vi "Fetch (Waveform).vi"(7 "Segment Index (0)":i32 format="%.0g", 8 "error in (no error)":errorcluster, 9 "Maximum Time (10000ms)":u32, 10 "Channel (1: Channel 1)":i32(ring) items=["Channel 1", "Channel 2", "Channel 3", "Channel 4", "Function 1", "Function 2", "Function 3", "Function 4", "Memory 1", "Memory 2", "Memory 3", "Memory 4"], 11 "VISA resource name":refnum<visa-resource-name>) -> (0 "error out":errorcluster, 2 "Waveform Data":waveform(dbl)(graph), 3 "VISA resource name out":refnum<visa-resource-name>)   [LabVIEW 2009, in "Agilent 8000 Series.lvlib"]
doc: "Returns the waveform the oscilloscope acquired for the specified channel. The waveform is from an acquisition that you initiate prior to calling this VI.\n\nYou use the Initiate VI to start an acquisition on the channels that you enable with the Configure Channel VI. The oscilloscope acquires waveforms for the enabled channels concurrently. You must call this VI separately for each enabled channel to obtain the waveforms.\n\nYou can call the Read Waveform VI instead of using low-level VIs.\n\n<B>Note:</B> Use this VI only with other low-level VIs. The high-level VIs automatically incorporate this functionality. This VI does not check the instrument status."
uses:
  Agilent 8000 Series.lvlib
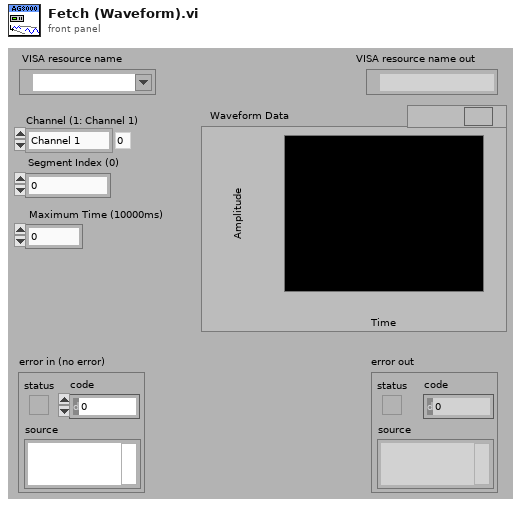
[diagram p1: front panel]
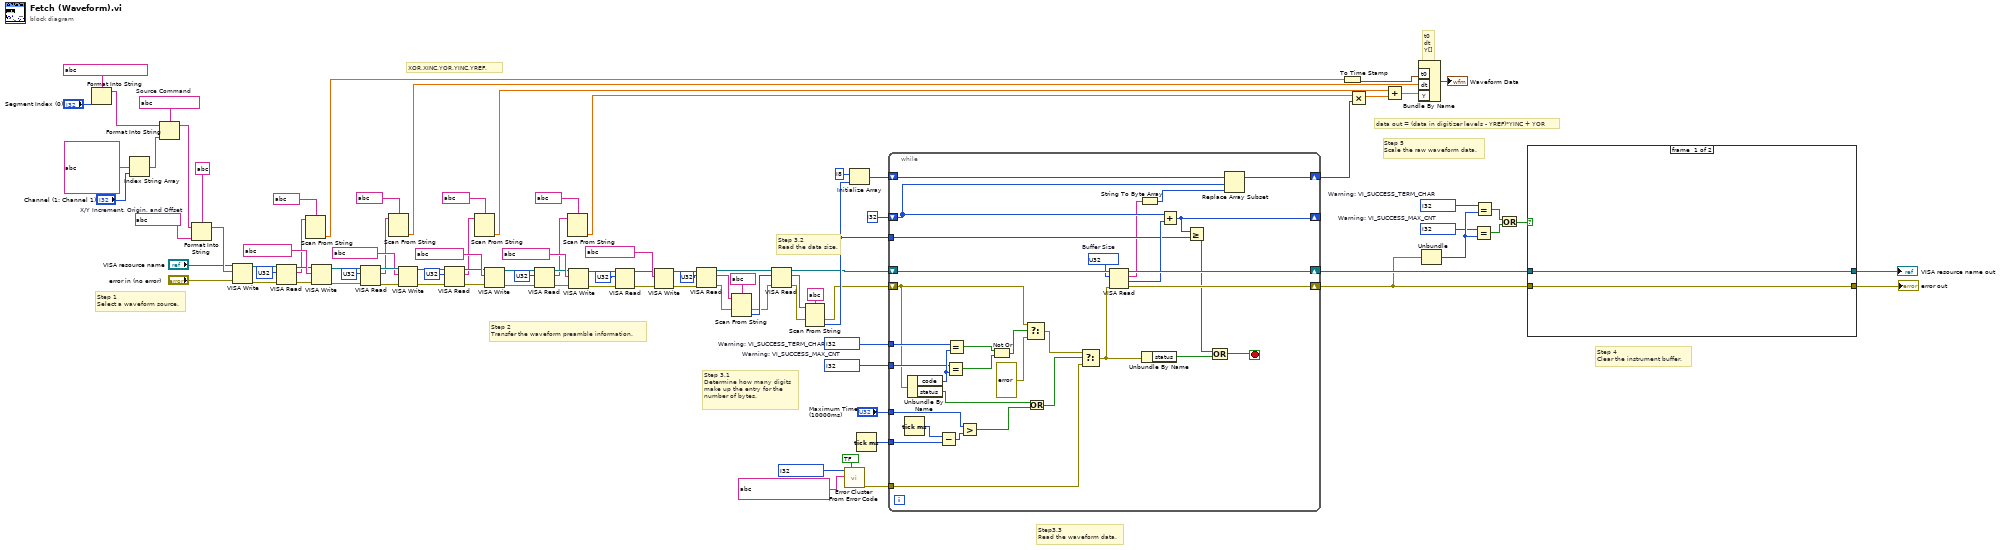
[diagram p0: block diagram]
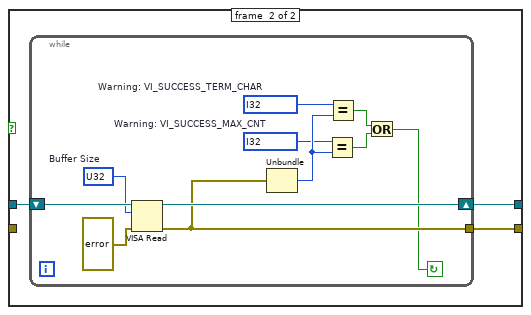
[diagram p2: hidden frame]
diagram:
  w69 = i32 ?  # Warning: VI_SUCCESS_MAX_CNT
  w68 = i32 ?  # Warning: VI_SUCCESS_TERM_CHAR
  w61 = i32 ?  # Warning: VI_SUCCESS_MAX_CNT
  w60 = i32 ?  # Warning: VI_SUCCESS_TERM_CHAR
  w91 = string ?  # Source Command
  w82 = string ?  # X/Y Increment, Origin, and Offset
  # "Step 5    \nScale the raw waveform data."
  # "Step 4    \nClear the instrument buffer."
  # "Step3.3   \nRead the waveform data."
  # "Step 3.2     \nRead the data size."
  # "Step 3.1     \nDetermine how many digits\nmake up the entry for the \nnumber of bytes."
  # "Step 2\nTransfer the waveform preamble information."
  # "Step 1       \nSelect a waveform source."
  # "XOR,XINC,YOR,YINC,YREF,"
  # "data out = (data in digitizer levels - YREF)*YINC + YOR"
  # "t0\ndt\nY[]"
  n1 = Format Into String(format string=string ?, "Segment Index (0)") -> (resulting string=w77:string)  [unwired: 2 in, 1 out]
  n2 = Index String Array(1:"Channel (1: Channel 1)", 2:string[] ?) -> (0:w83:string)  [unwired: 1 in]
  n3 = Format Into String(format string=w91, initial string=w77, w83) -> (resulting string=w89:string)  [unwired: 1 in, 1 out]
  n4 = Format Into String(format string=string ?, initial string=w89, w82) -> (resulting string=w88:string)  [unwired: 1 in, 1 out]
  n5 = VISA Write(VISA resource name="VISA resource name", write buffer=w88, error in (no error)="error in (no error)") -> (VISA resource name out=w96:refnum<visa-resource-name>, error out=w95:errorcluster)  [unwired: 1 out]
  n6 = VISA Read(VISA resource name=w96, byte count=u32 ?, error in (no error)=w95) -> (VISA resource name out=w31:refnum<visa-resource-name>, read buffer=w8:string, error out=w30:errorcluster)  [unwired: 1 out]
  n7 = Scan From String(format string=string ?, input string=w8) -> (output 1=w4:dbl)  [unwired: 3 in, 3 out]
  n8 = VISA Write(VISA resource name=w31, write buffer=string ?, error in (no error)=w30) -> (VISA resource name out=w29:refnum<visa-resource-name>, error out=w28:errorcluster)  [unwired: 1 out]
  n9 = VISA Read(VISA resource name=w29, byte count=u32 ?, error in (no error)=w28) -> (VISA resource name out=w27:refnum<visa-resource-name>, read buffer=w7:string, error out=w26:errorcluster)  [unwired: 1 out]
  n10 = Scan From String(format string=string ?, input string=w7) -> (output 1=w3:dbl)  [unwired: 3 in, 3 out]
  n11 = VISA Write(VISA resource name=w27, write buffer=string ?, error in (no error)=w26) -> (VISA resource name out=w25:refnum<visa-resource-name>, error out=w24:errorcluster)  [unwired: 1 out]
  n12 = VISA Read(VISA resource name=w25, byte count=u32 ?, error in (no error)=w24) -> (VISA resource name out=w23:refnum<visa-resource-name>, read buffer=w6:string, error out=w22:errorcluster)  [unwired: 1 out]
  n13 = Scan From String(format string=string ?, input string=w6) -> (output 1=w2:dbl)  [unwired: 3 in, 3 out]
  n14 = VISA Write(VISA resource name=w23, write buffer=string ?, error in (no error)=w22) -> (VISA resource name out=w21:refnum<visa-resource-name>, error out=w20:errorcluster)  [unwired: 1 out]
  n15 = VISA Read(VISA resource name=w21, byte count=u32 ?, error in (no error)=w20) -> (VISA resource name out=w19:refnum<visa-resource-name>, read buffer=w5:string, error out=w18:errorcluster)  [unwired: 1 out]
  n16 = Scan From String(format string=string ?, input string=w5) -> (output 1=w1:dbl)  [unwired: 3 in, 3 out]
  n17 = VISA Write(VISA resource name=w19, write buffer=string ?, error in (no error)=w18) -> (VISA resource name out=w17:refnum<visa-resource-name>, error out=w16:errorcluster)  [unwired: 1 out]
  n18 = VISA Read(VISA resource name=w17, byte count=u32 ?, error in (no error)=w16) -> (VISA resource name out=w15:refnum<visa-resource-name>, error out=w14:errorcluster)  [unwired: 2 out]
  n19 = VISA Write(VISA resource name=w15, write buffer=string ?, error in (no error)=w14) -> (VISA resource name out=w44:refnum<visa-resource-name>, error out=w43:errorcluster)  [unwired: 1 out]
  n20 = VISA Read(VISA resource name=w44, byte count=u32 ?, error in (no error)=w43) -> (VISA resource name out=w50:refnum<visa-resource-name>, read buffer=w47:string, error out=w46:errorcluster)  [unwired: 1 out]
  n21 = Scan From String(format string=string ?, input string=w47, error in=w46) -> (error out=w49:errorcluster, output 1=w76:i32)  [unwired: 2 in, 2 out]
  n22 = VISA Read(VISA resource name=w50, byte count=w76, error in (no error)=w49) -> (VISA resource name out=w54:refnum<visa-resource-name>, read buffer=w53:string, error out=w51:errorcluster)  [unwired: 1 out]
  n23 = Scan From String(format string=string ?, input string=w53, error in=w51) -> (error out=w55:errorcluster, output 1=w59:i32)  [unwired: 2 in, 2 out]
  n24 = call <vilib>:"Error Cluster From Error Code.vi"("show call chain? (False)"=bool ?, "error message (\"\")"=string ? ("error message (\"\")"), "error code (0)"=i32 ?) -> ("error out"=w67:errorcluster)  [unwired: 6 in]
  n25 = Initialize Array(i8 ? ("element"), w59) -> (w57:i8[])
  n26 = Tick Count (ms)() -> (millisecond timer value=w66:u32)
  n27 = while {
    shift-right: [w124] -> w74
    shift-left: w55 -> [w111]
    shift-right: [w129] -> w75
    shift-left: w54 -> [w128]
    shift-right: [w125] -> w39
    shift-left: w57 -> [w126]
    shift-right: [w121] -> _
    shift-left: i32 ? ("index") -> [w122]
    tunnel: w59 -> [w120]
    tunnel: w60 -> [w113]
    tunnel: w61 -> [w112]
    tunnel: "Maximum Time (10000ms)" -> [w108]
    tunnel: w66 -> [w107]
    tunnel: w67 -> [w102]
    stop <- w99 stop-if-true
    w127 = u32 ?  # Buffer Size
    n28 = Tick Count (ms)() -> (millisecond timer value=w109:u32)
    n29 = Unbundle By Name(w111) -> ("code"=w114:i32, "status"=w106:bool)
    n30 = Subtract(x=w109, y=w107) -> (x-y=w110:u32)
    n31 = Equal?(x=w112, y=w114) -> (x = y?=w117:bool)
    n32 = Equal?(x=w113, y=w114) -> (x = y?=w118:bool)
    n33 = Greater?(x=w108, y=w110) -> (0:w105:bool)
    n34 = Not Or(1:w117, 2:w118) -> (0:w116:bool)
    n35 = Select(t=w111, s=w116, f=errorcluster ? ("error in (no error)")) -> (s? t:f=w104:errorcluster)
    n36 = Or(x=w106, y=w105) -> (x .or. y?=w103:bool)
    n37 = Select(t=w104, s=w103, f=w102) -> (s? t:f=w101:errorcluster)
    n38 = VISA Read(VISA resource name=w128, byte count=w127, error in (no error)=w101) -> (VISA resource name out=w129:refnum<visa-resource-name>, read buffer=w98:string, return count=w123:u32, error out=w124:errorcluster)
    n39 = String To Byte Array(string=w98) -> (unsigned byte array=w97:u8[])
    n40 = Unbundle By Name(w101) -> ("status"=w100:bool)
    n41 = Add(x=w122, y=w123) -> (x+y=w121:u32)
    n42 = Greater Or Equal?(x=w121, y=w120) -> (x >= y?=w119:bool)
    n43 = Compound Arithmetic op=OR(w119, w100) -> (w99:bool)
    n44 = Replace Array Subset(array=w126, new element=w97, index=w122) -> (w125:i8[])
  }
  n45 = To Time Stamp(1:w4) -> (0:w93:timestamp)
  n46 = Multiply(x=w1, y=w39) -> (x*y=w86:dbl[])
  n47 = Add(x=w2, y=w86) -> (x+y=w87:dbl[])
  n48 = Bundle By Name("t0"=w93, "dt"=w3, "Y"=w87) -> (→"Waveform Data":waveform(dbl))  [unwired: 1 in]
  n49 = Unbundle(w74) -> ("code"=w70:i32)  [unwired: 2 out]
  n50 = Equal?(x=w69, y=w70) -> (x = y?=w72:bool)
  n51 = Equal?(x=w68, y=w70) -> (x = y?=w73:bool)
  n52 = Or(x=w73, y=w72) -> (x .or. y?=w71:bool)
  n53 = case shown="True" w71 {
    tunnel: w75 -> [w131 w134]
    tunnel: w74 -> [w130 _]
    tunnel: [w131 w133] -> w41
    tunnel: [w130 w132] -> w40
    frame #0 {
    }
    frame #1 {
      n54 = while {
        shift-right: [w144] -> w133
        shift-left: w134 -> [w145]
        tunnel: [w137] -> w132
        stop <- w136 continue-if-true
        w139 = i32 ?  # Warning: VI_SUCCESS_MAX_CNT
        w138 = i32 ?  # Warning: VI_SUCCESS_TERM_CHAR
        w143 = u32 ?  # Buffer Size
        n55 = VISA Read(VISA resource name=w145, byte count=w143, error in (no error)=errorcluster ?) -> (VISA resource name out=w144:refnum<visa-resource-name>, error out=w137:errorcluster)  [unwired: 2 out]
        n56 = Unbundle(w137) -> ("code"=w140:i32)  [unwired: 2 out]
        n57 = Equal?(x=w139, y=w140) -> (x = y?=w141:bool)
        n58 = Equal?(x=w138, y=w140) -> (x = y?=w142:bool)
        n59 = Or(x=w142, y=w141) -> (x .or. y?=w136:bool)
      }
    }
  }
  "error out" <- w40
  "VISA resource name out" <- w41
